vi "Begin.vi"(11 "Image Size":T1=enum."320x240") -> (0 "error out":errorcluster)   [LabVIEW 2013]
doc: "Called before other user functions, this VI is expected to open initial I/O refnums, load in file data, and do all program initialization. Notice that the <B>error out</B> terminal is simply used for data flow. Wiring it to other structures or subVIs ensures that this VI runs first."
uses:
  <vilib>/Rock Robotics/WPI/Camera/WPI_CameraImageSize.ctl
  <vilib>/Rock Robotics/WPI/Camera/WPI_CameraWhite Balance Values.ctl
  <vilib>/Rock Robotics/WPI/Camera/WPI_CameraExposure Values.ctl
  <vilib>/Rock Robotics/WPI/Camera/WPI_CameraFrameRate.ctl
  <vilib>/Rock Robotics/WPI/SafetyOutput/WPI_SafetyOutputConfigMenu.ctl
  <vilib>/Rock Robotics/WPI/DriverStation/WPI_DriverStationRobotMode2.ctl
  <vilib>/Rock Robotics/WPI/Joystick/WPI_JoystickDeviceEnum.ctl
  <vilib>/Rock Robotics/SystemInterfaces/DIO/FPGA_DIOPWMChannel.ctl
  <vilib>/Rock Robotics/SystemInterfaces/AI/FPGA_AIGyroChannel.ctl
  <vilib>/Rock Robotics/WPI/Solenoid/WPI_SolenoidChannel.ctl
  <vilib>/Rock Robotics/SystemInterfaces/Typedef/FPGA_TypedefSolenoidModule.ctl
  <vilib>/Rock Robotics/SystemInterfaces/DIO/FPGA_DIOChannel.ctl
  <vilib>/Rock Robotics/SystemInterfaces/AI/FPGA_AIChannel.ctl
  Robot Global Data.vi
  <vilib>/Rock Robotics/WPI/RobotDrive/WPI_RobotDriveOpen4MotorWithTalon.vi
  <vilib>/Rock Robotics/WPI/Solenoid/WPI_SolenoidOpenSingle.vi
  <vilib>/Rock Robotics/WPI/MotorControl/WPI_MotorControlOpen Victor.vi
  <vilib>/Rock Robotics/WPI/Counter/WPI_CounterDigitalInputToDigitalSource.vi
  <vilib>/Rock Robotics/WPI/Counter/WPI_CounterOpen Gear Tooth Sensor Mode.vi
panel:
  in  "Gain (VoltsPerDegree/Second)":dbl=0.007
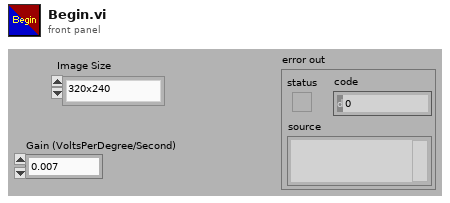
[diagram p1: front panel]
types:
  T1 = typedef "WPI_CameraImageSize.ctl" = enum16{"640x480", "320x240", "160x120"}
  T2 = typedef "FPGA_DIOChannel.ctl" = enum8{"DIO 1", "DIO 2", "DIO 3", "DIO 4", "DIO 5", "DIO 6", "DIO 7", "DIO 8", "DIO 9", "DIO 10", "DIO 11", "DIO 12", "DIO 13", "DIO 14", "Invalid"}
  T3 = typedef "FPGA_DIOPWMChannel.ctl" = enum8{"PWM 1", "PWM 2", "PWM 3", "PWM 4", "PWM 5", "PWM 6", "PWM 7", "PWM 8", "PWM 9", "PWM 10", "Invalid"}
  T4 = typedef "FPGA_AIChannel.ctl" = enum8{"AI 1", "AI 2", "AI 3", "AI 4", "AI 5", "AI 6", "AI 7", "AI 8", "Invalid"}
  T5 = typedef "FPGA_TypedefSolenoidModule.ctl" = enum16{"Solenoid Module 1", "Solenoid Module 2"}
  T6 = typedef "WPI_SolenoidChannel.ctl" = enum8{"Solenoid 1", "Solenoid 2", "Solenoid 3", "Solenoid 4", "Solenoid 5", "Solenoid 6", "Solenoid 7", "Solenoid 8", "Invalid"}
  T7 = typedef "FPGA_AIGyroChannel.ctl" = enum8{"AI 1", "AI 2", "Invalid"}
  T8 = typedef "WPI_JoystickDeviceEnum.ctl" = enum16{"USB 1", "USB 2", "USB 3", "USB 4", "Kinect 1", "Kinect 2"}
  T9 = typedef "WPI_DriverStationRobotMode2.ctl" = enum16{"Autonomous Disabled", "Autonomous Enabled", "Teleop Disabled", "Teleop Enabled", "Timeout", "Finish", "Test Disabled", "Test Enabled"}
  T10 = typedef "WPI_SafetyOutputConfigMenu.ctl" = enum16{"Enable", "Disable"}
  T11 = typedef "WPI_CameraFrameRate.ctl" = u32
  T12 = typedef "WPI_CameraExposure Values.ctl" = enum16{"Auto", "Flicker-free 50 Hz", "Flicker-free 60 Hz", "Hold current"}
  T13 = typedef "WPI_CameraWhite Balance Values.ctl" = enum16{"Auto", "Fixed indoor", "Fixed outdoor 1", "Fixed outdoor 2", "Fixed fluorescent 1", "Fixed fluorescent 2", "Hold current"}
  T14 = typedef "WPI_GyroDevRef.ctl" = cluster{"DevStatus":errorcluster, "Analog Module":T15, "Analog Channel":T4, "Offset":dbl, "Gain (VoltsPerDegree/Second)":dbl}
  T15 = typedef "FPGA_TypedefAnalogModule.ctl" = enum16{"Analog Module 1", "Analog Module 2"}
  T16 = typedef "WPI_AnalogChannelDevRef.ctl" = cluster{"DevStatus":errorcluster, "Analog Module":T15, "Analog Channel":T4}
  T17 = typedef "WPI_JoystickDevRef.ctl" = cluster{"Device":T8}
  T18 = typedef "WPI_CameraDevRef.ctl" = cluster{"Camera Address":string, "CameraStatus":errorcluster, "Acquire Image Notifier":refnum<notifier>}
  T19 = typedef "WPI_RobotDriveDevRef.ctl" = cluster{"DevStatus":errorcluster, "Motors[]":T20[], "Square Inputs":bool, "Max Output":dbl, "Isochronous":bool}
  T20 = typedef "WPI_MotorControlDeviceRef.ctl" = cluster{"DeviceStatus":errorcluster, "Type":enum16{"PWM", "CAN"}, "PWM":cluster{"Digital Module":T21, "PWM Channel":T3, "DeadBand":T22}, "CAN":cluster{"Device Number":u8, "Control Mode":T23, "Semaphore":T24, "Max Vout":dbl}, "Invert":bool, "TransformRef":T25, "InvTransformRef":T25}
  T21 = typedef "FPGA_TypedefDigitalModule.ctl" = enum16{"Digital Module 1", "Digital Module 2"}
  T22 = typedef "WPI_PWMDeadband.ctl" = cluster{"Name":string, "maxPositivePwm":i32, "minPositivePwm":i32, "centerPwm":i32, "maxNegativePwm":i32, "minNegativePwm":i32, "angularRange":u16}
  T23 = typedef "WPI_CANJaguar_ControlMode.ctl" = enum8{"Percent VBus", "Current", "Speed", "Position", "Voltage"}
  T24 = typedef "Semaphore RefNum" = refnum<k1>
  T25 = typedef "WPI_PWMTransform_ConPane.ctl" = refnum<vi>
  T26 = typedef "WPI_DigitalInputDevRef.ctl" = cluster{"DevStatus":errorcluster, "DIO Channel":T2, "Digital Module":T21}
  T27 = typedef "FPGA_CounterEncoderSourceConvertionLVSourceType.ctl" = cluster{"DevStatus":errorcluster, "AnalogTriggerMode?":bool, "DigitalMode":cluster{"Digital Module":T21, "DIO Channel":T28}, "AnalogTriggerMode":cluster{"AnalogTriggerIndex":T29, "OutputType":T30}}
  T28 = typedef "FPGA_DIODigitalSourceChannel.ctl" = enum8{"DIO 1", "DIO 2", "DIO 3", "DIO 4", "DIO 5", "DIO 6", "DIO 7", "DIO 8", "DIO 9", "DIO 10", "DIO 11", "DIO 12", "DIO 13", "DIO 14", "Disabled"}
  T29 = typedef "FPGA_AnalogTriggerIndex.ctl" = enum8{"Trig 0", "Trig 1", "Trig 2", "Trig 3", "Trig 4", "Trig 5", "Trig 6", "Trig 7", "Invalid"}
  T30 = typedef "FPGA_AnalogTriggerOutType.ctl" = enum16{"InWindow", "TriggerState", "Rising", "Falling"}
  T31 = typedef "WPI_CounterDevRef.ctl" = cluster{"DevStatus":errorcluster, "CntIndex":T32}
  T32 = typedef "FPGA_CounterCtrSystemIndex.ctl" = enum8{"Ctr 0", "Ctr 1", "Ctr 2", "Ctr 3", "Ctr 4", "Ctr 5", "Ctr 6", "Ctr 7", "Invalid"}
  T33 = typedef "WPI_SolenoidDevRef.ctl" = cluster{"DevStatus":errorcluster, "Solenoid Module":T5, "Forward Solenoid Channel":T6, "Reverse Solenoid Channel":T6}
  T34 = typedef "WPI_ServoDeviceRef.ctl" = cluster{"DeviceStatus":errorcluster, "Digital Module":T21, "PWM Channel":T3, "DeadBand":T22}
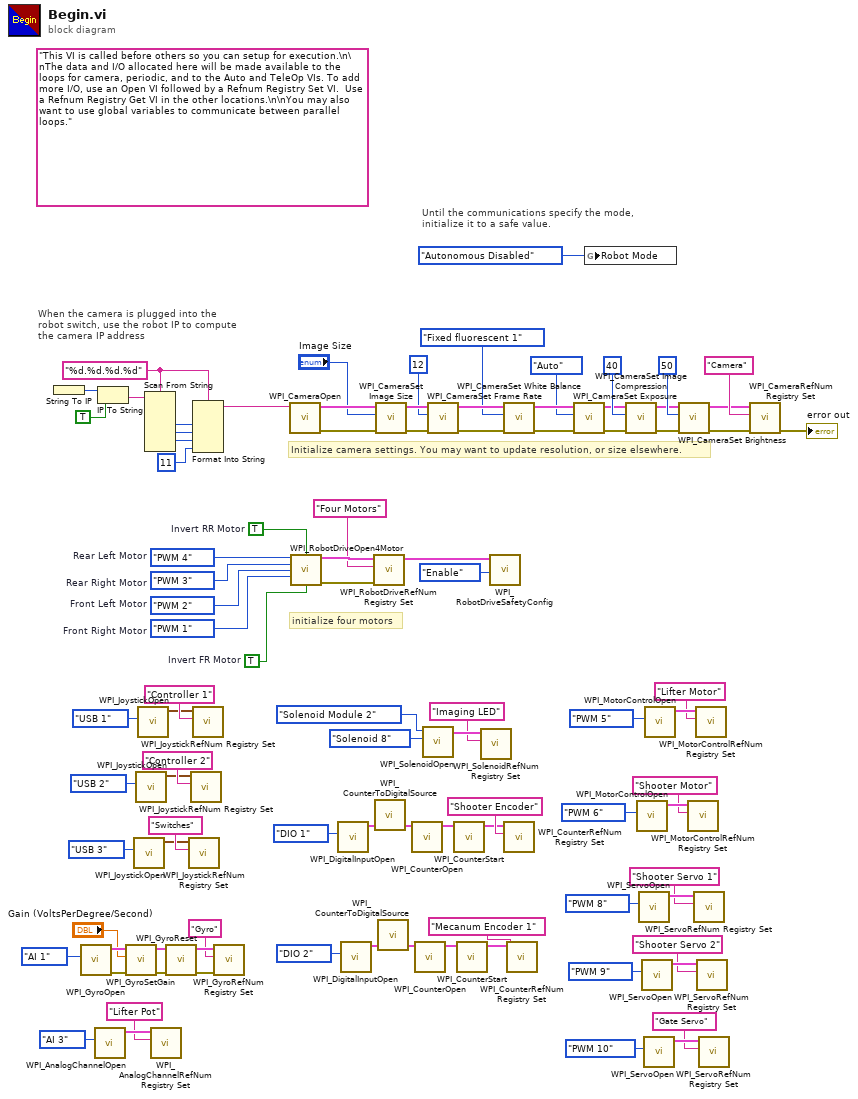
[diagram p0: block diagram]
diagram:
  w51 = TRUE  # Invert FR Motor
  w10 = TRUE  # Invert RR Motor
  w52 = FPGA_DIOPWMChannel."PWM 1"  # Front Right Motor
  w53 = FPGA_DIOPWMChannel."PWM 2"  # Front Left Motor
  w54 = FPGA_DIOPWMChannel."PWM 3"  # Rear Right Motor
  w55 = FPGA_DIOPWMChannel."PWM 4"  # Rear Left Motor
  w64 = "%d.%d.%d.%d" ("format string")
  (unwired) "This VI is called before others so you can setup for execution.\n\nThe data and I/O allocated here will be made available to the loops for camera, periodic, and to the Auto and TeleOp VIs. To add more I/O, use an Open VI followed by a Refnum Registry Set VI.  Use a Refnum Registry Get VI in the other locations.\n\nYou may also want to use global variables to communicate between parallel loops."
  # "Until the communications specify the mode,\ninitialize it to a safe value."
  # "When the camera is plugged into the\nrobot switch, use the robot IP to compute\nthe camera IP address"
  # "initialize four motors"
  # "Initialize camera settings. You may want to update resolution, or size elsewhere."
  n1 = String To IP() -> (0:w71:u32)  [unwired: 1 in]
  n2 = call <vilib>:"WPI_GyroOpen.vi"("Analog Channel"=FPGA_AIGyroChannel."AI 1") -> ("error out"=w40:errorcluster, "GyroDevRef"=w42:T14)  [unwired: 5 in, 4 out]
  n3 = call <vilib>:"WPI_AnalogChannelOpen.vi"("Analog Channel"=FPGA_AIChannel."AI 3") -> ("AIDeviceRef"=w12:T16)  [unwired: 9 in, 1 out]
  n4 = IP To String(1:TRUE ("dot notation? (F)"), 2:w71) -> (0:w69:string)
  n5 = call <vilib>:"WPI_GyroSetGain.vi"("error in (no error)"=w40, "Gain (VoltsPerDegree/Second)"="Gain (VoltsPerDegree/Second)", "GyroDevRef"=w42) -> ("error out"=w44:errorcluster, "GyroDevRef"=w43:T14)  [unwired: 7 out]
  n6 = call <vilib>:"WPI_JoystickOpen.vi"("JoystickDevice"=WPI_JoystickDeviceEnum."USB 3") -> ("JoystickDevRef"=w46:T17)  [unwired: 10 in]
  n7 = call <vilib>:"WPI_JoystickOpen.vi"("JoystickDevice"=WPI_JoystickDeviceEnum."USB 2") -> ("JoystickDevRef"=w49:T17)  [unwired: 10 in]
  n8 = call <vilib>:"WPI_JoystickOpen.vi"("JoystickDevice"=WPI_JoystickDeviceEnum."USB 1") -> ("JoystickDevRef"=w58:T17)  [unwired: 10 in]
  n9 = Scan From String(format string=w64, input string=w69) -> (output 1=w68:i32, output 2=w67:i32, output 3=w66:i32)  [unwired: 7 in, 3 out]
  n10 = call <vilib>:"WPI_AnalogChannelRefNum Registry Set.vi"("refnum name"="Lifter Pot", "AIDeviceRef"=w12) -> ()  [unwired: 8 in, 2 out]
  n11 = call <vilib>:"WPI_GyroReset.vi"("error in (no error)"=w44, "GyroDevRef"=w43) -> ("error out"=w38:errorcluster, "GyroDevRef"=w37:T14)  [unwired: 8 out]
  n12 = call <vilib>:"WPI_JoystickRefNum Registry Set.vi"("refnum name"="Switches", "JoystickDevRef"=w46) -> ()  [unwired: 8 in, 2 out]
  n13 = call <vilib>:"WPI_JoystickRefNum Registry Set.vi"("refnum name"="Controller 2", "JoystickDevRef"=w49) -> ()  [unwired: 8 in, 2 out]
  n14 = Format Into String(format string=w64, w68, w67, w66, 11 ("Compression")) -> (resulting string=w60:string)  [unwired: 2 in, 1 out]
  n15 = call <vilib>:"WPI_JoystickRefNum Registry Set.vi"("refnum name"="Controller 1", "JoystickDevRef"=w58) -> ()  [unwired: 8 in, 2 out]
  n16 = call <vilib>:"WPI_GyroRefNum Registry Set.vi"("error in (no error)"=w38, "refnum name"="Gyro", "GyroDevRef"=w37) -> ()  [unwired: 7 in, 2 out]
  n17 = call <vilib>:"WPI_CameraOpen.vi"("Camera Address"=w60) -> ("error out"=w83:errorcluster, "CameraDevRef"=w84:T18)  [unwired: 2 in, 7 out]
  n18 = call-poly <vilib>:"WPI_RobotDriveOpen4Motor.vi"("Rear Left Motor"=w55, "Rear Right Motor Inverted"=w10, "Rear Right Motor"=w54, "Front Left Motor"=w53, "Front Right Motor"=w52, "Front Right Motor Inverted"=w51) -> ("RobotDriveDevRef"=w94:T19, "error out"=w92:errorcluster)  [unwired: 8 in]
  n19 = call <vilib>:"WPI_DigitalInputOpen.vi"("DIO Channel"=FPGA_DIOChannel."DIO 1") -> ("DigitalInputDevRef"=w25:T26)  [unwired: 9 in, 1 out]
  n20 = call <vilib>:"WPI_DigitalInputOpen.vi"("DIO Channel"=FPGA_DIOChannel."DIO 2") -> ("DigitalInputDevRef"=w6:T26)  [unwired: 9 in, 1 out]
  n21 = call <vilib>:"WPI_RobotDriveRefNum Registry Set.vi"("error in (no error)"=w92, "refnum name"="Four Motors", "RobotDriveDevRef"=w94) -> ("RobotDriveDevRef"=w63:T19)  [unwired: 8 out]
  n22 = call-poly <vilib>:"WPI_CounterToDigitalSource.vi"("DigitalInputDevRef"=w25) -> ("Digital Source"=w24:T27)  [unwired: 6 in]
  n23 = call <vilib>:"WPI_CameraSet Image Size.vi"("error in (no error)"=w83, "Image Size"="Image Size", "CameraDevRef"=w84) -> ("error out"=w82:errorcluster, "CameraDevRef Out"=w85:T18)  [unwired: 7 out]
  n24 = call-poly <vilib>:"WPI_CounterToDigitalSource.vi"("DigitalInputDevRef"=w6) -> ("Digital Source"=w5:T27)  [unwired: 6 in]
  n25 = call-poly <vilib>:"WPI_CounterOpen.vi"("Source"=w24) -> ("CounterDevRef"=w21:T31)  [unwired: 9 in, 1 out]
  n26 = call-poly <vilib>:"WPI_CounterOpen.vi"("Source"=w5) -> ("CounterDevRef"=w2:T31)  [unwired: 9 in, 1 out]
  n27 = call-poly <vilib>:"WPI_SolenoidOpen.vi"("Solenoid Channel"=WPI_SolenoidChannel."Solenoid 8", "Solenoid Module (Module 1)"=FPGA_TypedefSolenoidModule."Solenoid Module 2") -> ("SolenoidDevRef"=w33:T33)  [unwired: 1 in, 8 out]
  n28 = call <vilib>:"WPI_CameraSet Frame Rate.vi"("error in (no error)"=w82, "Frame Rate (fps)"=T11 12, "CameraDevRef"=w85) -> ("error out"=w81:errorcluster, "CameraDevRef Out"=w87:T18)  [unwired: 7 out]
  n29 = call <vilib>:"WPI_CounterStart.vi"("CounterDevRef in"=w21) -> ("CounterDevRef out"=w20:T31)  [unwired: 9 in, 1 out]
  n30 = call <vilib>:"WPI_CounterStart.vi"("CounterDevRef in"=w2) -> ("CounterDevRef out"=w1:T31)  [unwired: 9 in, 1 out]
  n31 = call <vilib>:"WPI_SolenoidRefNum Registry Set.vi"("refnum name"="Imaging LED", "SolenoidDevRef"=w33) -> ()  [unwired: 8 in, 2 out]
  n32 = call <vilib>:"WPI_RobotDriveSafetyConfig.vi"("mode"=WPI_SafetyOutputConfigMenu."Enable", "RobotDriveDevRef"=w63) -> ()  [unwired: 8 in, 2 out]
  n33 = call <vilib>:"WPI_CameraSet White Balance.vi"("error in (no error)"=w81, "White Balance"=WPI_CameraWhite_Balance_Values."Fixed fluorescent 1", "CameraDevRef"=w87) -> ("error out"=w80:errorcluster, "CameraDevRef Out"=w86:T18)  [unwired: 7 out]
  n34 = call <vilib>:"WPI_CounterRefNum Registry Set.vi"("refnum name"="Shooter Encoder", "CounterDevRef"=w20) -> ()  [unwired: 8 in, 2 out]
  n35 = call <vilib>:"WPI_CounterRefNum Registry Set.vi"("refnum name"="Mecanum Encoder 1", "CounterDevRef"=w1) -> ()  [unwired: 8 in, 2 out]
  n36 = call <vilib>:"WPI_CameraSet Exposure.vi"("error in (no error)"=w80, "Exposure"=WPI_CameraExposure_Values."Auto", "CameraDevRef"=w86) -> ("error out"=w79:errorcluster, "CameraDevRef Out"=w89:T18)  [unwired: 7 out]
  n37 = global write "Robot Global Data.vi" "Robot Mode"(WPI_DriverStationRobotMode2."Autonomous Disabled" ("Robot Mode")) -> ()
  n38 = call <vilib>:"WPI_CameraSet Image Compression.vi"("error in (no error)"=w79, "Compression"=40, "CameraDevRef"=w89) -> ("error out"=w78:errorcluster, "CameraDevRef Out"=w88:T18)  [unwired: 7 out]
  n39 = call-poly <vilib>:"WPI_MotorControlOpen.vi"("PWM Channel"=FPGA_DIOPWMChannel."PWM 6") -> ("MotorControlDeviceRef"=w27:T20)  [unwired: 6 in, 4 out]
  n40 = call <vilib>:"WPI_ServoOpen.vi"("PWM Channel"=FPGA_DIOPWMChannel."PWM 8") -> ("ServoDeviceRef"=w9:T34)  [unwired: 9 in, 1 out]
  n41 = call <vilib>:"WPI_ServoOpen.vi"("PWM Channel"=FPGA_DIOPWMChannel."PWM 9") -> ("ServoDeviceRef"=w31:T34)  [unwired: 9 in, 1 out]
  n42 = call <vilib>:"WPI_ServoOpen.vi"("PWM Channel"=FPGA_DIOPWMChannel."PWM 10") -> ("ServoDeviceRef"=w19:T34)  [unwired: 9 in, 1 out]
  n43 = call-poly <vilib>:"WPI_MotorControlOpen.vi"("PWM Channel"=FPGA_DIOPWMChannel."PWM 5") -> ("MotorControlDeviceRef"=w15:T20)  [unwired: 6 in, 4 out]
  n44 = call <vilib>:"WPI_CameraSet Brightness.vi"("error in (no error)"=w78, "Brightness"=50, "CameraDevRef"=w88) -> ("error out"=w76:errorcluster, "CameraDevRef Out"=w77:T18)  [unwired: 7 out]
  n45 = call <vilib>:"WPI_MotorControlRefNum Registry Set.vi"("refnum name"="Shooter Motor", "MotorControlDevRef"=w27) -> ()  [unwired: 8 in, 2 out]
  n46 = call <vilib>:"WPI_ServoRefNum Registry Set.vi"("refnum name"="Shooter Servo 1", "ServoDeviceRef"=w9) -> ()  [unwired: 8 in, 2 out]
  n47 = call <vilib>:"WPI_MotorControlRefNum Registry Set.vi"("refnum name"="Lifter Motor", "MotorControlDevRef"=w15) -> ()  [unwired: 8 in, 2 out]
  n48 = call <vilib>:"WPI_ServoRefNum Registry Set.vi"("refnum name"="Shooter Servo 2", "ServoDeviceRef"=w31) -> ()  [unwired: 8 in, 2 out]
  n49 = call <vilib>:"WPI_ServoRefNum Registry Set.vi"("refnum name"="Gate Servo", "ServoDeviceRef"=w19) -> ()  [unwired: 8 in, 2 out]
  n50 = call <vilib>:"WPI_CameraRefNum Registry Set.vi"("error in (no error)"=w76, "refnum name"="Camera", "CameraDevRef"=w77) -> ("error out"=→"error out":errorcluster)  [unwired: 8 out]
